vi "Voltage - Velocity.vi"() -> ()   [LabVIEW 2018]
doc: "This example demonstrates how to continuously acquire buffered voltage measurements using a DAQmx device.\n\nFor instructions on how to connect your signals to the DAQ device, refer to your device documentation."
uses:
  <vilib>/Utility/error.llb/DialogType.ctl
  <vilib>/DAQmx/read.llb/DAQmx Read (Analog 1D Wfm NChan NSamp).vi
  <vilib>/DAQmx/create/channels.llb/DAQmx Create Channel (AI-Voltage-Basic).vi
  <vilib>/DAQmx/configure/timing.llb/DAQmx Timing (Sample Clock).vi
  <vilib>/DAQmx/miscellaneous.llb/DAQmx Fill In Error Info.vi
  <resource>/objmgr/daqmx.rc
panel:
  out "Waveform Chart":waveform(dbl)[](graph)
  in  "Stop":bool
  out "Waveform Graph":waveform(dbl)[](graph)
  in  "Number of Samples":i32=100
  in  "Sample Rate":dbl=1000.0
  in  "Sample Clock Source":tag="OnboardClock"
  out "Actual Sample Rate":dbl=1000.0 format="%0.2f"
  # "Channel Settings"
  # "Acquired Data"
  # "Timing Settings"
  # "Trigger Settings"
  # "Logging Settings"
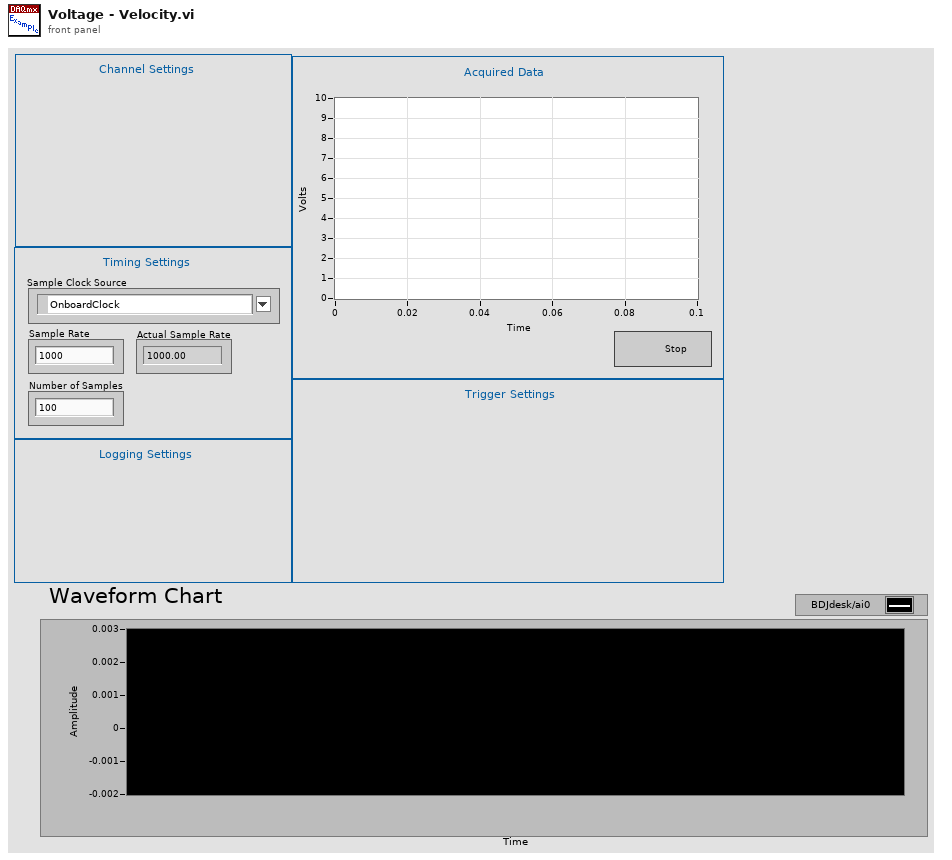
[diagram p1: front panel]
types:
  T1 = typedef "DialogType.ctl" = u16
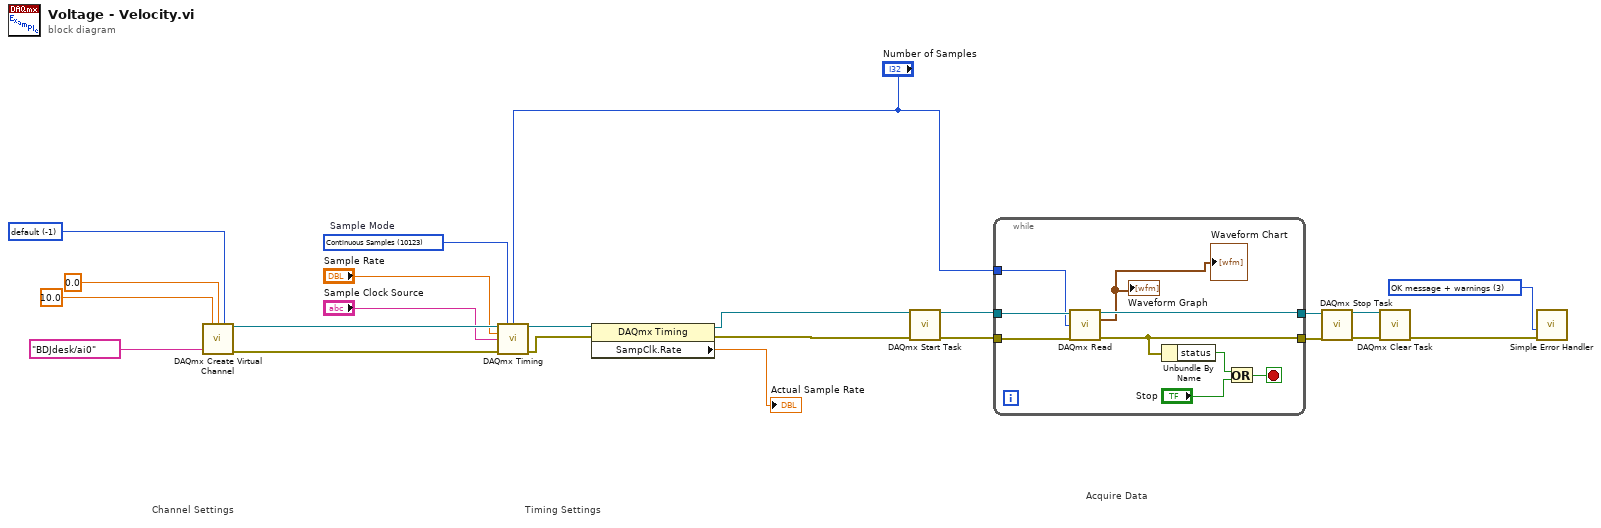
[diagram p0: block diagram]
diagram:
  w11 = -1 items=["default"=-1, "RSE"=10083, "NRSE"=10078, "Differential"=10106, "Pseudodifferential"=12529] ("Terminal Configuration")
  w1 = T1 3 items=["no dialog", "OK message", "continue or stop message", "OK message + warnings", "continue/stop + warnings"] ("type of dialog (OK msg:1)")
  w21 = 10123 items=["Finite Samples"=10178, "Continuous Samples"=10123, "Hardware Timed Single Point"=12522]  # Sample Mode
  # "Acquire Data"
  # "Timing Settings"
  # "Channel Settings"
  n1 = call-poly <vilib>:"DAQmx Create Virtual Channel.vi"("maximum value"=10.0 ("Max Voltage"), "minimum value"=0.0 ("Min Voltage"), "input terminal configuration"=w11, "physical channels"=tag "BDJdesk/ai0" ("Physical Channel")) -> ("task out"=w19:refnum<k21>, "error out"=w20:errorcluster)  [unwired: 10 in]
  n2 = call-poly <vilib>:"DAQmx Timing.vi"("task/channels in"=w19, "sample mode"=w21, "samples per channel"="Number of Samples", "rate"="Sample Rate", "source"="Sample Clock Source", "error in"=w20) -> ("task out"=w23:refnum<k21>, "error out"=w22:errorcluster)  [unwired: 8 in]
  n3 = property class="DAQmx Timing"(reference=w23, error in=w22) -> (reference out=w18:refnum<k21>, error out=w17:errorcluster, "SampClk.Rate"=→"Actual Sample Rate":dbl)
  n4 = call <vilib>:"DAQmx Start Task.vi"("task/channels in"=w18, "error in"=w17) -> ("task out"=w16:refnum<k21>, "error out"=w15:errorcluster)  [unwired: 12 in]
  n5 = while {
    tunnel: w16 -> [w32]
    tunnel: w15 -> [w31]
    tunnel: [w30] -> w5
    tunnel: [w28] -> w4
    tunnel: "Number of Samples" -> [w25]
    stop <- w26 stop-if-true
    n6 = call-poly <vilib>:"DAQmx Read.vi"("task/channels in"=w32, "number of samples per channel"=w25, "error in"=w31) -> ("task out"=w30:refnum<k21>, "data"=→"Waveform Graph" →"Waveform Chart":waveform(dbl)[], "error out"=w28:errorcluster)  [unwired: 10 in]
    n7 = Unbundle By Name(w28) -> ("status"=w27:bool)
    n8 = Or(x=w27, y="Stop") -> (x .or. y?=w26:bool)
  }
  n9 = call <vilib>:"DAQmx Stop Task.vi"("task/channels in"=w5, "error in"=w4) -> ("task out"=w2:refnum<k21>, "error out"=w3:errorcluster)  [unwired: 12 in]
  n10 = call <vilib>:"DAQmx Clear Task.vi"("task in"=w2, "error in"=w3) -> ("error out"=w14:errorcluster)  [unwired: 13 in]
  n11 = call <vilib>:"Simple Error Handler.vi"("type of dialog (OK msg:1)"=w1, "error in (no error)"=w14) -> ()  [unwired: 3 in, 5 out]
